vi "DHE_DRV_support_abort_read.vi"(5 "support abort?":bool, 11 "error in (no error)":errorcluster) -> (4 "fd out":i32, 8 "return value":i32, 15 "error out":errorcluster)   [LabVIEW 2016]
doc: "This VI closes the I/O interface with the instrument."
uses:
  c/lib/libarcDHE.so
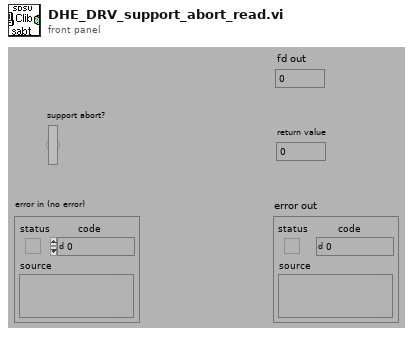
[diagram p1: front panel]
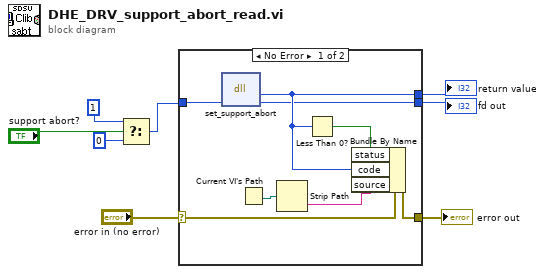
[diagram p0: block diagram]
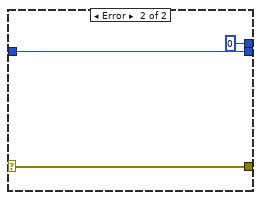
[diagram p2: hidden frame]
diagram:
  n1 = Select(t=1, s="support abort?", f=0) -> (s? t:f=w1:i32)
  n2 = case shown="No Error" "error in (no error)" {
    selector: "error in (no error)" -> [w9 w17]
    tunnel: w1 -> [w16 w19]
    tunnel: [w14 0] -> w8
    tunnel: [w11 w17] -> w7
    tunnel: [w10 w19] -> w6
    frame No Error {
      n3 = dll-call lib="home/simager/panview/PAN/Modules/SDSU/private/c/lib/libarcDHE.so" fn="set_support_abort" label="support abort read"("sabt"=w16) -> (w14:i32, "sabt"=w10:u16)  [unwired: 3 in, 2 out]
      n4 = Current VI's Path() -> (path=w13:path)
      n5 = Strip Path(path=w13) -> (name=w12:string)  [unwired: 1 out]
      n6 = Less Than 0?(x=w14) -> (x < 0?=w15:bool)
      n7 = Bundle By Name(cluster=w9, "status"=w15, "code"=w14, "source"=w12) -> (w11:errorcluster)
    }
    frame Error {
    }
  }
  "error out" <- w7
  "return value" <- w8
  "fd out" <- w6
